vi "add channel to configuration.vi"(8 "error in":errorcluster, 10 "channel":refnum<class "TBM channel.lvclass">, 11 "sample module configuration in":refnum<class "sample module configuration.lvclass">) -> (0 "error out":errorcluster, 3 "sample module configuration out":refnum<class "sample module configuration.lvclass">)   [LabVIEW 2013, in "sample module configuration.lvclass"]
doc: "Adds a single channel to the configuration"
uses:
  sample module configuration.lvclass
  channel/TBM channel.lvclass
  sample module configuration.lvclass/sample module configuration.ctl
  <vilib>/NI/Tag Bus/tag/tag descriptor.lvclass/tag descriptor.ctl
  <vilib>/NI/Tag Bus/tag/tag descriptor.lvclass
  root configuration/TBM configuration.lvclass
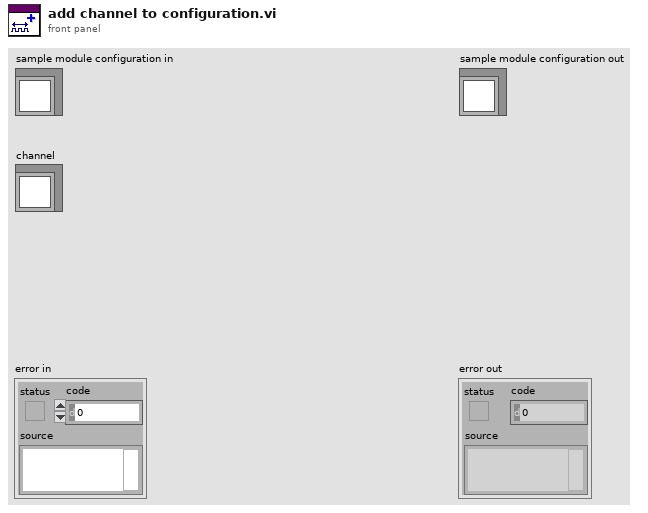
[diagram p1: front panel]
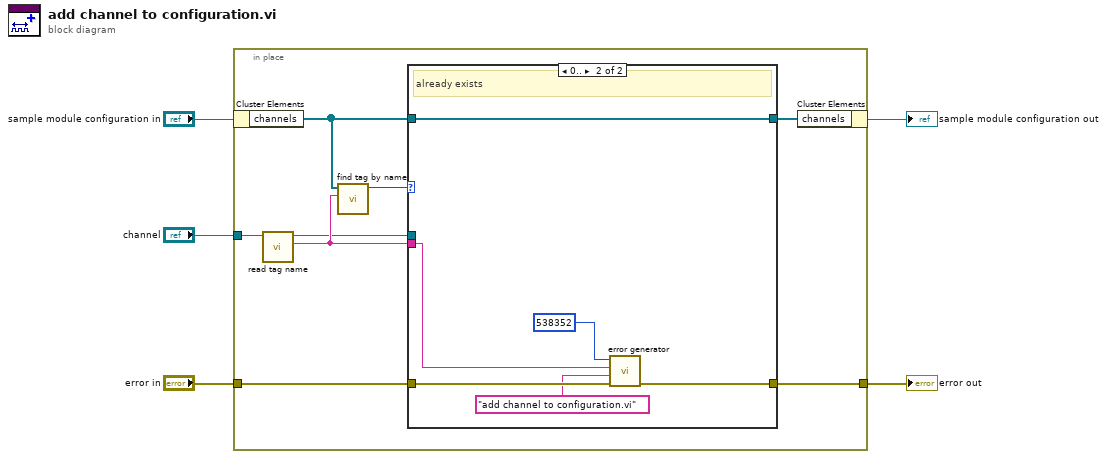
[diagram p0: block diagram]
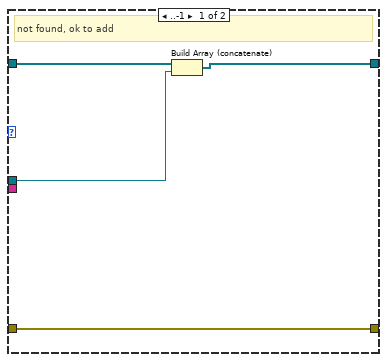
[diagram p2: hidden frame]
diagram:
  n1 = in-place {
    in-place-border: "channel" -> [w13]
    in-place-border: "error in" -> [w11]
    in-place-border: [w8] -> w1
    n2 = in-place-cluster #1("sample module configuration in") -> ("channels"=w6:refnum<class "TBM channel.lvclass">[])
    n3 = call <vilib>:"read tag name.vi"("system tag in"=w13) -> ("name"=w10:string, "system tag out"=w9:refnum<class "TBM channel.lvclass">)  [unwired: 8 in, 1 out]
    n4 = call <vilib>:"find tag by name.vi"("name"=w10, "tags in"=w6) -> ("index"=w12:i32)  [unwired: 9 in]
    n5 = case shown="0.." w12 {
      tunnel: w11 -> [w14 w23]
      tunnel: w10 -> [_ w20]
      tunnel: w9 -> [w15 _]
      tunnel: w6 -> [w17 w19]
      tunnel: [w14 w22] -> w8
      tunnel: [w16 w19] -> w7
      frame ..-1 {
        # "not found, ok to add"
        n6 = Build Array (concatenate)(w17, w15) -> (w16:refnum<class "TBM channel.lvclass">[])
      }
      frame 0.. {
        # "already exists"
        n7 = call "error generator.vi"("error in"=w23, "source"="add channel to configuration.vi", "append error message"=w20, "error code (0)"=538352) -> ("error out"=w22:errorcluster)  [unwired: 7 in]
      }
    }
    n8 = in-place-cluster #1("channels"=w7) -> (→"sample module configuration out":refnum<class "sample module configuration.lvclass">)
  }
  "error out" <- w1
